vi "test class filtering.vi"() -> ()   [LabVIEW 2013, in "NISE_CEF_Tests.lvlib"]
uses:
  NISE_CEF_Tests.lvlib
  Trunk/Configuration Framework/serializable node/NISE_CEF_serializable node.lvclass
  Trunk/ProjectTemplates/Source/Advanced Configurator/Classes/channel node/channel node.lvclass
  Trunk/ProjectTemplates/Source/Advanced Configurator/Classes/cRIO node/cRIO  node root.lvclass
  Trunk/ProjectTemplates/Source/Configuration Editor Framework/Classes/cRIO/cRIO.lvclass
  Trunk/ProjectTemplates/Source/Configuration Editor Framework/Classes/Channel/Channel.lvclass
  Trunk/Configuration Framework/Node/NISE_CEF_Node.lvclass
panel:
  out "OK":bool
  out "no err":errorcluster
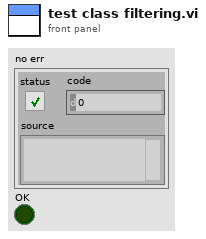
[diagram p1: front panel]
types:
  T1 = typedef "NISE_CEF_Node.lvclass/NodeRef.ctl" = refnum<data-value>
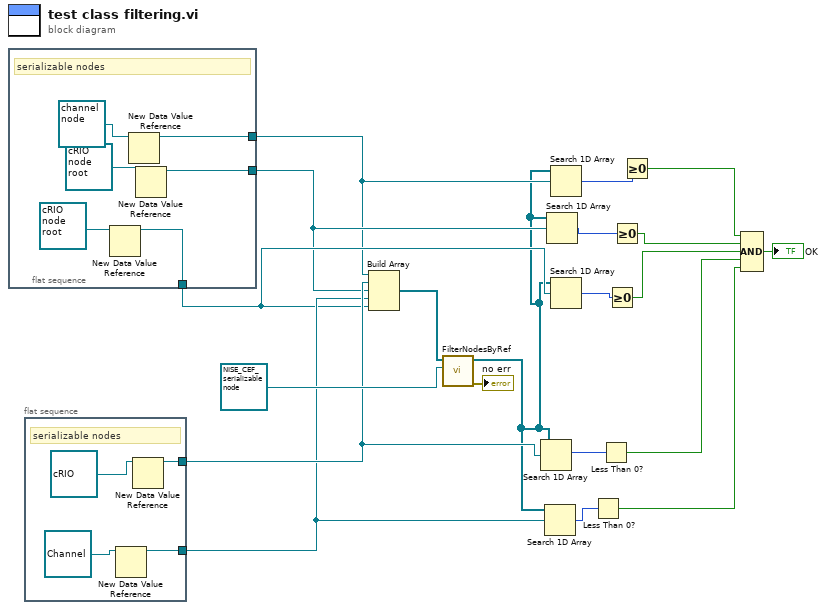
[diagram p0: block diagram]
diagram:
  n1 = flat-sequence {
    tunnel: [w23] -> w13
    tunnel: [w22] -> w14
    tunnel: [w21] -> w15
    frame #0 {
      # "serializable nodes"
      n2 = New Data Value Reference(data value=refnum<class "cRIO  node root.lvclass"> refnum ("cRIO  node root.lvclass")) -> (data value reference=w21:refnum<data-value>)  [unwired: 1 in, 1 out]
      n3 = New Data Value Reference(data value=refnum<class "channel node.lvclass"> refnum ("channel node.lvclass")) -> (data value reference=w23:refnum<data-value>)  [unwired: 1 in, 1 out]
      n4 = New Data Value Reference(data value=refnum<class "cRIO  node root.lvclass"> refnum ("cRIO  node root.lvclass")) -> (data value reference=w22:refnum<data-value>)  [unwired: 1 in, 1 out]
    }
  }
  n5 = flat-sequence {
    tunnel: [w28] -> w17
    tunnel: [w27] -> w16
    frame #0 {
      # "serializable nodes"
      n6 = New Data Value Reference(data value=refnum<class "Channel.lvclass"> refnum ("Channel.lvclass")) -> (data value reference=w27:refnum<data-value>)  [unwired: 1 in, 1 out]
      n7 = New Data Value Reference(data value=refnum<class "cRIO.lvclass"> refnum ("cRIO.lvclass")) -> (data value reference=w28:refnum<data-value>)  [unwired: 1 in, 1 out]
    }
  }
  n8 = Build Array(w13, w17, w14, w16, w15) -> (w19:refnum<data-value>[])
  n9 = call "FilterNodesByRef.vi"("NISE_CEF_Node"=refnum<class "NISE_CEF_serializable node.lvclass"> refnum ("NISE_CEF_serializable node.lvclass"), "nodes"=w19) -> ("error out"=→"no err":errorcluster, "filtered nodes"=w1:T1[])  [unwired: 8 in]
  n10 = Search 1D Array(1D array=w1, element=w17) -> (index of element=w9:i32)  [unwired: 1 in]
  n11 = Search 1D Array(1D array=w1, element=w16) -> (index of element=w8:i32)  [unwired: 1 in]
  n12 = Search 1D Array(1D array=w1, element=w14) -> (index of element=w11:i32)  [unwired: 1 in]
  n13 = Search 1D Array(1D array=w1, element=w13) -> (index of element=w10:i32)  [unwired: 1 in]
  n14 = Search 1D Array(1D array=w1, element=w15) -> (index of element=w12:i32)  [unwired: 1 in]
  n15 = Less Than 0?(x=w8) -> (x < 0?=w7:bool)
  n16 = Less Than 0?(x=w9) -> (x < 0?=w6:bool)
  n17 = Greater Or Equal To 0?(x=w12) -> (x >= 0?=w5:bool)
  n18 = Greater Or Equal To 0?(x=w11) -> (x >= 0?=w4:bool)
  n19 = Greater Or Equal To 0?(x=w10) -> (x >= 0?=w3:bool)
  n20 = Compound Arithmetic op=AND(w3, w4, w5, w6, w7) -> (→"OK":bool)
